vi "Open Handle.vi"(6 "verify server(true)":bool=TRUE, 7 "cookie file":path, 8 "error in (no error)":errorcluster, 9 "password":string, 10 "username":string, 11 "HTTP Client reqwest in":refnum<class "HTTP Client reqwest.lvclass">) -> (0 "error out":errorcluster, 3 "HTTP Client reqwest out":refnum<class "HTTP Client reqwest.lvclass">)   [LabVIEW 2021, in "HTTP Client reqwest.lvclass"]
uses:
  HTTP Client reqwest.lvclass
  HTTP Client reqwest.lvclass/HTTP Client reqwest.ctl
  external/reqwest-rs-labview/lv_src/ClientBuilder/ClientBuilder.lvclass
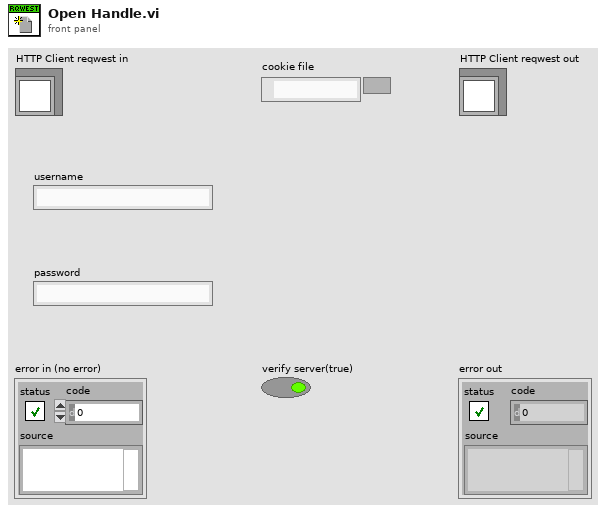
[diagram p1: front panel]
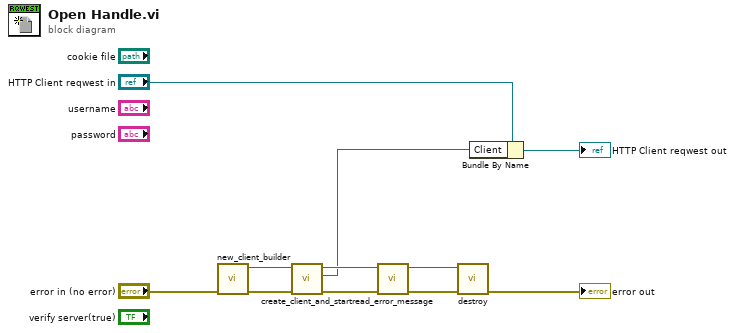
[diagram p0: block diagram]
diagram:
  n1 = call "new_client_builder.vi"("error in (no error)"="error in (no error)") -> ("error out"=w10:errorcluster, "Client out"=w11:refnum<class "ClientBuilder.lvclass">)  [unwired: 9 in]
  n2 = call "create_client_and_start.vi"("error in"=w10, "ClientBuilder in"=w11) -> ("error out"=w7:errorcluster, "Client out"=w3:refnum<class "Client.lvclass">, "ClientBuilder out"=w9:refnum<class "ClientBuilder.lvclass">)  [unwired: 7 in]
  n3 = call "read_error_message.vi"("error in (no error)"=w7, "ClientBuilder in"=w9) -> ("error out"=w6:errorcluster, "ClientBuilder in"=w8:refnum<class "ClientBuilder.lvclass">)  [unwired: 7 in, 1 out]
  n4 = call "destroy.vi"("error in (no error)"=w6, "ClientBuilder in"=w8) -> ("error out"=→"error out":errorcluster)  [unwired: 9 in]
  n5 = Bundle By Name(cluster="HTTP Client reqwest in", "Client"=w3) -> (→"HTTP Client reqwest out":refnum<class "HTTP Client reqwest.lvclass">)
